vi "path_logics.vi"(7 "bool_Erase":bool, 8 "error in":errorcluster, 10 "path_Destin":path, 11 "path_Orig":path) -> (0 "error out":errorcluster, 3 "arr_copiedfiles":path[](array[path]))   [LabVIEW 2026]
doc: "This subVI is the core of the logics, it calls each functions to \n1) check origin folder and its files \n2) log reford the information\n3) check all files data creation\n4) copy files and delete"
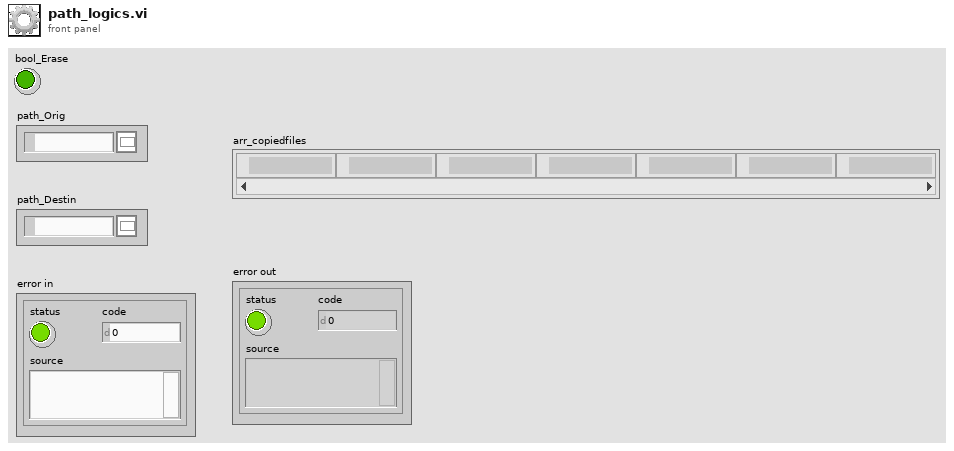
[diagram p1: front panel]
types:
  T1 = cluster{"path_Orig":path, "bo_Empty_Orig":bool, "bo_exist_Orig":bool, "path_Destin":path, "bo_Empty_Dest":bool, "bo_exist_Dest":bool, "bool_Erase":bool, "arr_cl_lastmod_path":cluster{"File Path":path, "DST":i32, "day of year":i32, "day of week":i32, "year":i32, "month":i32, "day of month":i32, "hour":i32, "minute":i32, "second":i32, "fractional second":dbl, "filename":string}[]}
  T2 = cluster{"filename":string, "arr_path out 2":path}[]
  T3 = cluster{"File Path":path, "DST":i32, "day of year":i32, "day of week":i32, "year":i32, "month":i32, "day of month":i32, "hour":i32, "minute":i32, "second":i32, "fractional second":dbl, "filename":string}[]
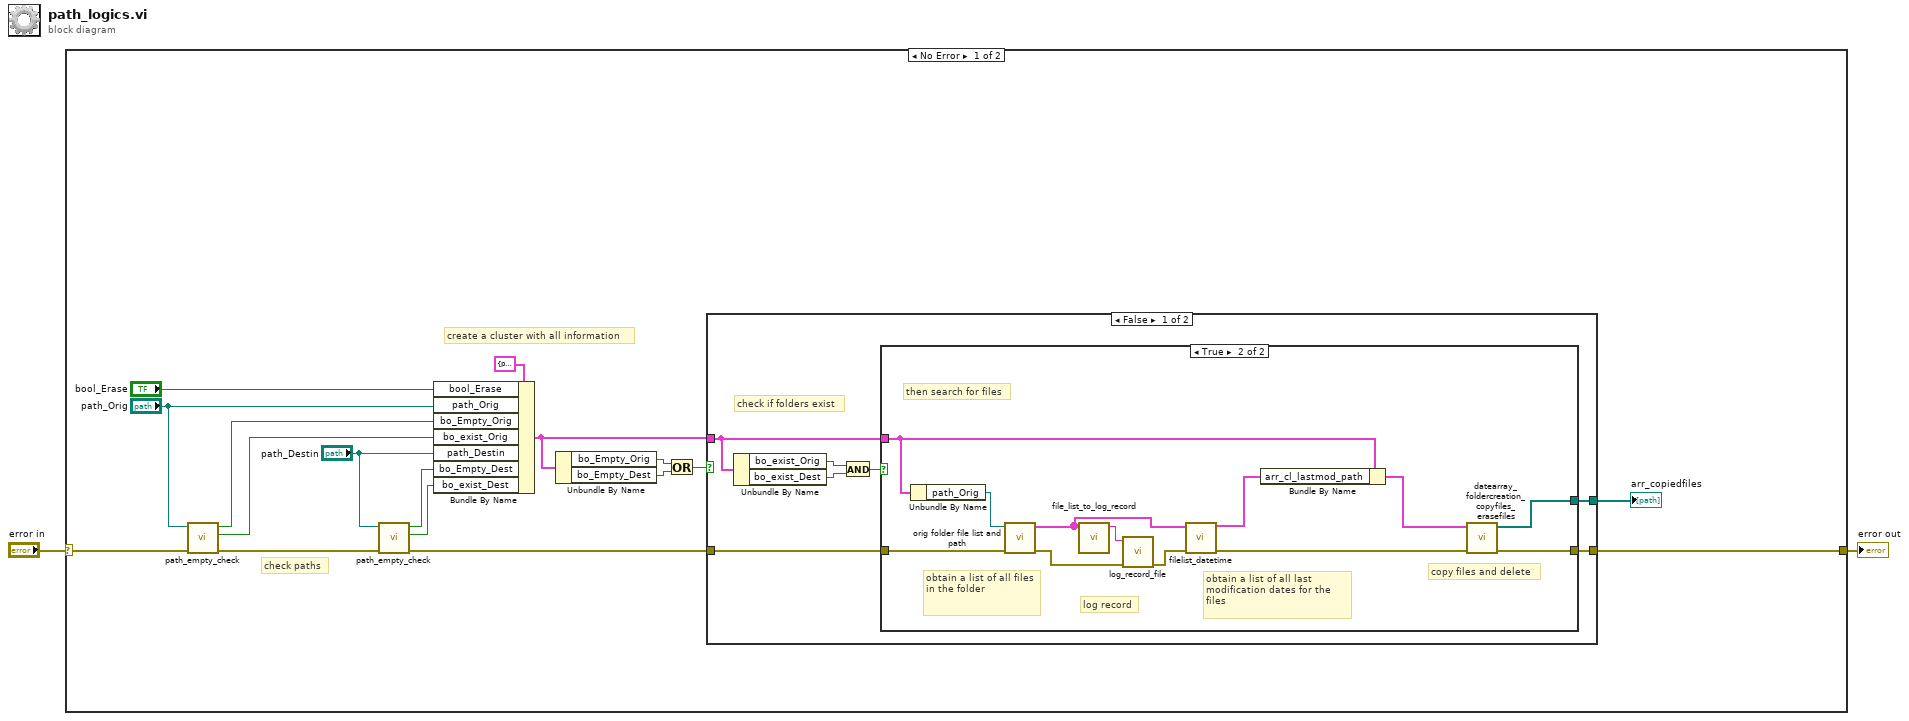
[diagram p0: block diagram]
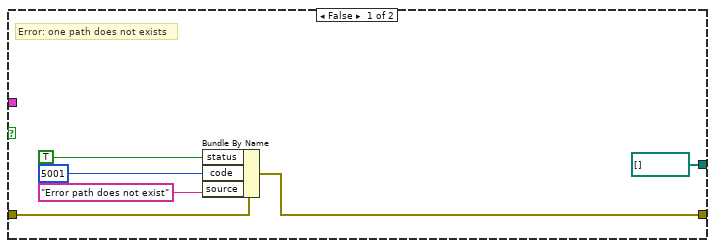
[diagram p2: hidden frame]
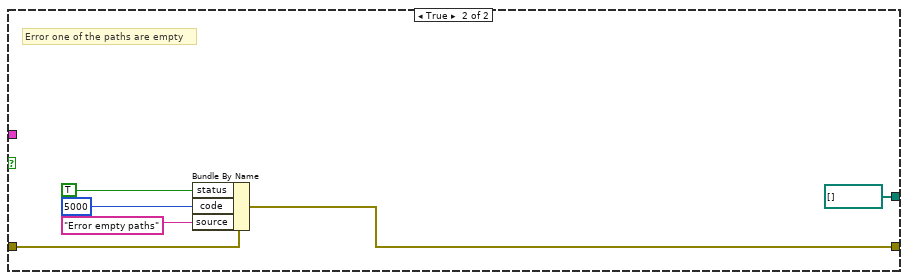
[diagram p3: hidden frame]
diagram:
  n1 = case shown="No Error" "error in" {
    selector: "error in" -> [w19 w51]
    tunnel: [w5 w51] -> w1
    frame No Error {
      # "check paths"
      # "create a cluster with all information"
      n2 = call "path_empty_check.vi"("error in"=w19, "path_Input"="path_Orig") -> ("error out"=w18:errorcluster, "bo_exist"=w14:bool, "bo_Empty"=w15:bool)  [unwired: 7 in]
      n3 = call "path_empty_check.vi"("error in"=w18, "path_Input"="path_Destin") -> ("error out"=w6:errorcluster, "bo_exist"=w11:bool, "bo_Empty"=w12:bool)  [unwired: 7 in]
      n4 = Bundle By Name(cluster=T1 {"path_Orig"=path "", "bo_Empty_Orig"=TRUE, "bo_exist_Orig"=TRUE, "path_Destin"=path "", "bo_Empty_Dest"=TRUE, "bo_exist_Dest"=TRUE, "bool_Erase"=FALSE, "arr_cl_lastmod_path"=[]}, "bool_Erase"="bool_Erase", "path_Orig"="path_Orig", "bo_Empty_Orig"=w15, "bo_exist_Orig"=w14, "path_Destin"="path_Destin", "bo_Empty_Dest"=w12, "bo_exist_Dest"=w11) -> (w10:T1)
      n5 = Unbundle By Name(w10) -> ("bo_Empty_Orig"=w9:bool, "bo_Empty_Dest"=w8:bool)
      n6 = Or(x=w9, y=w8) -> (x .or. y?=w7:bool)
      n7 = case shown="False" w7 {
        tunnel: w10 -> [w21 _]
        tunnel: w6 -> [w23 w50]
        tunnel: [w22 w49] -> w5
        tunnel: [w20 path[] [] ("arr_copiedfiles")] -> w3
        frame False {
          # "check if folders exist"
          n8 = Unbundle By Name(w21) -> ("bo_exist_Orig"=w25:bool, "bo_exist_Dest"=w24:bool)
          n9 = And(x=w25, y=w24) -> (x .and. y?=w26:bool)
          n10 = case shown="True" w26 {
            tunnel: w23 -> [w29 w40]
            tunnel: [w28 w42] -> w22
            tunnel: w21 -> [_ w44]
            tunnel: [path[] [] ("arr_copiedfiles") w33] -> w20
            frame False {
              # "Error: one path does not exists"
              n11 = Bundle By Name(cluster=w29, "status"=TRUE, "code"=5001, "source"="Error path does not exist") -> (w28:errorcluster)
            }
            frame True {
              # "log record"
              # "copy files and delete"
              # "obtain a list of all last modification dates for the files"
              # "obtain a list of all files in the folder"
              # "then search for files"
              n12 = Unbundle By Name(w44) -> ("path_Orig"=w41:path)
              n13 = call "orig folder file list and path.vi"("error in"=w40, "path_Orig"=w41) -> ("error out"=w39:errorcluster, "cl_filename_pathout"=w36:T2)  [unwired: 8 in]
              n14 = call "file_list_to_log_record.vi"("cl_filename_pathout"=w36) -> ("concatenated string"=w37:string)  [unwired: 10 in]
              n15 = call "log_record_file.vi"("error in"=w39, "st_LogEvent"=w37) -> ("error out"=w38:errorcluster)  [unwired: 9 in]
              n16 = call "filelist_datetime.vi"("error in"=w38, "cl_filename_pathout"=w36) -> ("error out"=w43:errorcluster, "arr_cl_lastmod_path"=w35:T3)  [unwired: 8 in]
              n17 = Bundle By Name(cluster=w44, "arr_cl_lastmod_path"=w35) -> (w34:T1)
              n18 = call "datearray_foldercreation_copyfiles_erasefiles.vi"("error in"=w43, "Cluster"=w34) -> ("error out"=w42:errorcluster, "arr_copiedfiles"=w33:path[])  [unwired: 8 in]
            }
          }
        }
        frame True {
          # "Error one of the paths are empty"
          n19 = Bundle By Name(cluster=w50, "status"=TRUE, "code"=5000, "source"="Error empty paths") -> (w49:errorcluster)
        }
      }
      "arr_copiedfiles" <- w3
    }
    frame Error {
    }
  }
  "error out" <- w1
